vi "camera testing.vi"() -> ()   [LabVIEW 2014]
uses:
  <vilib>/vision/Vision Builder AI/API.llb/IVB Interface - VBAI Version.ctl
  <vilib>/Instr/_visa.llb/VISA Configure Serial Port (Instr).vi
panel:
  out "y-position 3":dbl
  out "x-position 3":dbl
  out "y-position 2":dbl
  out "x-position 2":dbl
  out "y-position 1":dbl
  out "XY Graph":cluster{dbl[], dbl[]}(graph)
  out "x-position 1":dbl
  out "Velocity array":dbl[][](array[numeric])
  out "Position array":dbl[][](array[numeric]) format="%#_8g"
  in  "stop":bool
  # "y-pos"
  # "N"
  # "Time"
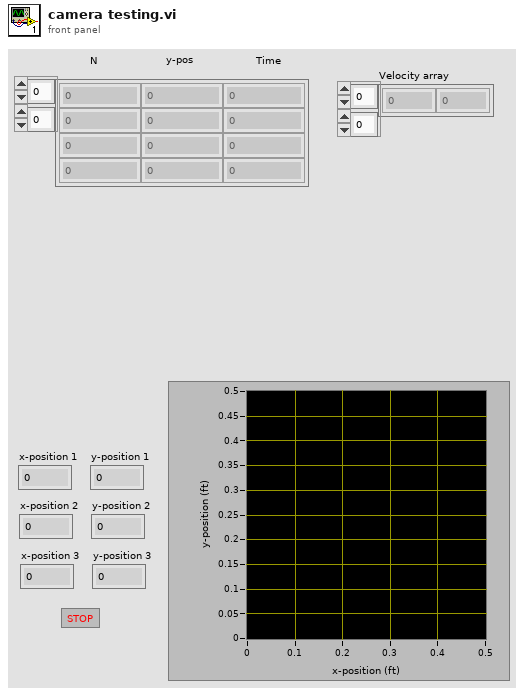
[diagram p1: front panel]
types:
  T1 = typedef "IVB Interface - VBAI Version.ctl" = u16
  T2 = typedef "VBAIInterface.ctl" = refnum<k21>
  T3 = typedef "IMAQ Image.ctl" = refnum<image>
  T4 = cluster{"PASS/FAIL Flag":bool, "Numeric Measurement":dbl, "String Measurement":string, "Report Text":string}[]
  T5 = cluster{"PASS/FAIL Flag":bool, "Numeric Measurement":dbl, "String Measurement":string, "Report Text":string}
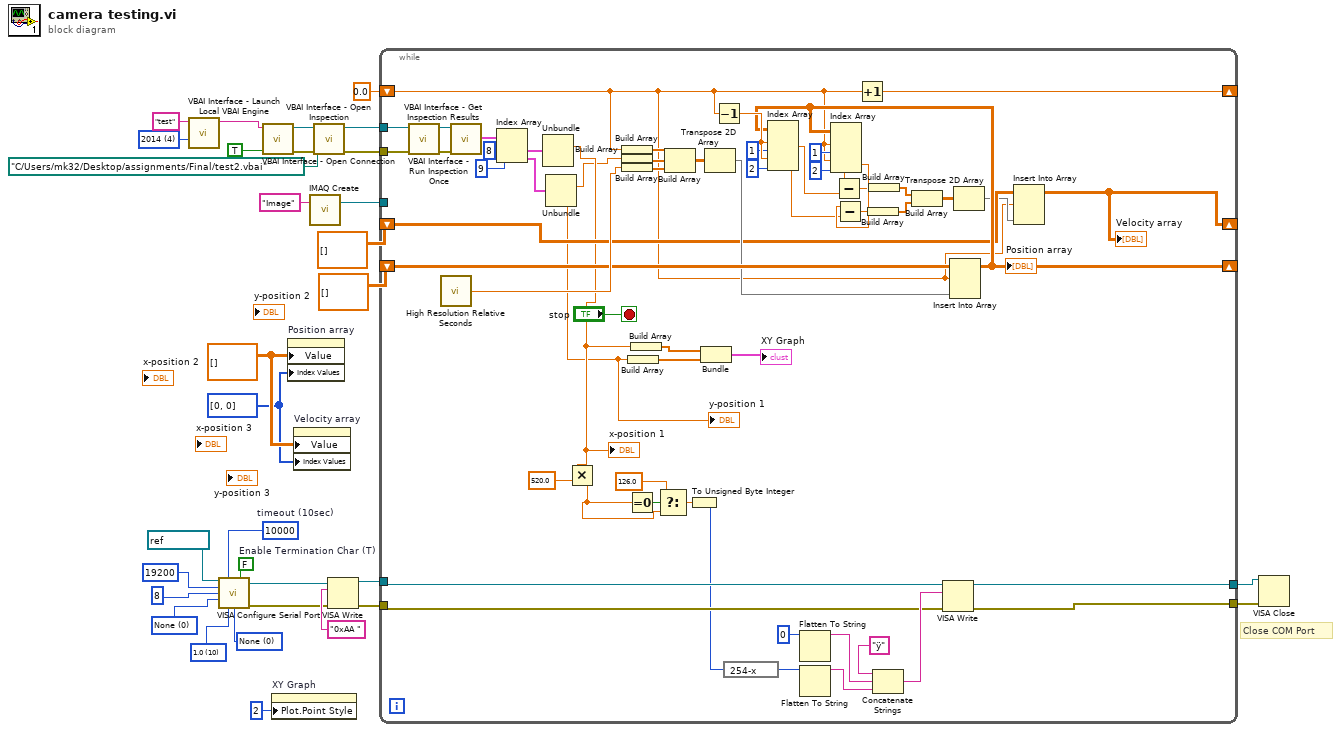
[diagram p0: block diagram]
diagram:
  w8 = u16 0 items=["None"=0, "XON/XOFF"=1, "RTS/CTS"=2, "DTR/DSR"=4] ("flow control")
  w9 = u16 10 items=["1.0"=10, "1.5"=15, "2.0"=20] ("stop bits")
  w10 = u16 0 items=["None", "Odd", "Even", "Mark", "Space"] ("parity")
  w14 = FALSE  # Enable Termination Char (T)
  w15 = u32 10000  # timeout (10sec)
  w18 = u32[] [0, 0] ("Index Values")
  w19 = dbl[][] [] ("output array")
  w28 = T1 4 items=["2010", "2011", "2012", "2013", "2014"] ("Engine Version")
  # "Close COM Port"
  n1 = call <vilib>:"VBAI Interface - Launch Local VBAI Engine.vi"("Engine Version"=w28, "Local VBAI Engine Name"="test") -> ("Session Name Out"=w29:string)  [unwired: 8 in, 1 out]
  n2 = call-poly "VISA Configure Serial Port"("VISA resource name"=refnum<visa-resource-name> "COM6", "timeout (10sec)"=w15, "Enable Termination\nChar (T)"=w14, "baud rate (9600)"=u32 19200 ("baud rate"), "data bits (8)"=u16 8 ("data bits"), "parity (0:none)"=w10, "stop bits (10: 1 bit)"=w9, "flow control (0:none)"=w8) -> ("VISA resource name out"=w6:refnum<visa-resource-name>, "error out"=w7:errorcluster)  [unwired: 1 in, 5 out]
  n3 = call <vilib>:"VBAI Interface - Open Connection.vi"("Force Connection (False)"=TRUE, "Session In"=w29) -> ("error out"=w27:errorcluster, "Session Out"=w26:T2)  [unwired: 8 in]
  n4 = property on="XY Graph" class="XYGraph (strict)"("Plot.Point Style"=u8 2) -> ()  [unwired: 2 in, 2 out]
  n5 = property on="Position array" class="Arr (strict)"("Value"=w19, "Index Values"=w18) -> ()  [unwired: 2 in, 2 out]
  n6 = property on="Velocity array" class="Arr (strict)"("Value"=w19, "Index Values"=w18) -> ()  [unwired: 2 in, 2 out]
  n7 = call "IMAQ Create"("Image Name"="Image") -> ("New Image"=w22:T3)  [unwired: 4 in, 1 out]
  n8 = call <vilib>:"VBAI Interface - Open Inspection.vi"("error in"=w27, "Path"=path "C:/Users/mk32/Desktop/assignments/Final/test2.vbai", "Session In"=w26) -> ("error out"=w23:errorcluster, "Session Out"=w24:T2)  [unwired: 7 in]
  n9 = VISA Write(VISA resource name=w6, write buffer="0xAA ", error in (no error)=w7) -> (VISA resource name out=w5:refnum<visa-resource-name>, error out=w4:errorcluster)  [unwired: 1 out]
  n10 = while {
    tunnel: w24 -> [w88]
    tunnel: w23 -> [w89]
    tunnel: w22 -> [_]
    shift-right: [w83] -> _
    shift-left: 0.0 ("Numeric Measurement") -> [w58]
    shift-right: [w61] -> _
    shift-left: dbl[][] [] ("appended array") -> [w77]
    shift-right: [w57] -> _
    shift-left: dbl[][] [] ("appended array") -> [w60]
    tunnel: w5 -> [w49]
    tunnel: w4 -> [w48]
    tunnel: [w47] -> w3
    tunnel: [w46] -> w2
    stop <- "stop" stop-if-true
    n11 = call <vilib>:"VBAI Interface - Run Inspection Once.vi"("error in"=w89, "Session In"=w88) -> ("error out"=w87:errorcluster, "Session Out"=w86:T2)  [unwired: 8 in]
    n12 = call <vilib>:"High Resolution Relative Seconds.vi"() -> ("relative seconds"=w82:dbl)
    n13 = call <vilib>:"VBAI Interface - Get Inspection Results.vi"("error in"=w87, "Session In"=w86) -> ("Step Results"=w85:T4)  [unwired: 3 in, 6 out]
    n14 = Index Array(array=w85, index #1=8 ("index"), index #2=9 ("index")) -> (element #1=w56:T5, element #2=w54:T5)
    n15 = Unbundle(w56) -> ("Numeric Measurement"=w41:dbl)  [unwired: 3 out]
    "x-position 1" <- w41
    n16 = Unbundle(w54) -> ("Numeric Measurement"=w33:dbl)  [unwired: 3 out]
    "y-position 1" <- w33
    n17 = Multiply(x=w41, y=520.0) -> (x*y=w39:dbl)
    n18 = Build Array(w58) -> (w81:dbl[])
    n19 = Build Array(w33) -> (w80:dbl[])
    n20 = Build Array(w82) -> (w79:dbl[])
    n21 = Equal To 0?(x=w39) -> (x = 0?=w42:bool)
    n22 = Build Array(w33) -> (w45:dbl[])
    n23 = Build Array(w41) -> (w44:dbl[])
    n24 = Select(t=126.0, s=w42, f=w39) -> (s? t:f=w36:dbl)
    n25 = Build Array(w81, w80, w79) -> (w78:dbl[][])
    n26 = To Unsigned Byte Integer(number=w36) -> (unsigned 8bit integer=w35:u8)
    n27 = Bundle(w44, w45) -> (→"XY Graph":cluster{dbl[], dbl[]})  [unwired: 1 in]
    n28 = Transpose 2D Array(2D array=w78) -> (transposed array=w62:dbl[][])
    n29 = Decrement(x=w58) -> (x-1=w76:dbl)
    n30 = expression code="254-x"(w35) -> (w34:u8)
    n31 = Flatten To String(anything=u8 0 ("y")) -> (data string=w52:string)  [unwired: 1 in, 4 out]
    n32 = Flatten To String(anything=w34) -> (data string=w51:string)  [unwired: 1 in, 4 out]
    n33 = Increment(x=w58) -> (x+1=w83:dbl)
    n34 = Concatenate Strings("ÿ", w52, w51) -> (w50:string)
    n35 = VISA Write(VISA resource name=w49, write buffer=w50, error in (no error)=w48) -> (VISA resource name out=w47:refnum<visa-resource-name>, error out=w46:errorcluster)  [unwired: 1 out]
    n36 = Insert Into Array(array=w77, index (row)=w58, new element=w62) -> (w61:dbl[][])  [unwired: 1 in]
    "Position array" <- w61
    n37 = Index Array(array=w61, index (row) #1=w76, index (col) #1=1 ("disabled index (col)"), index (row) #2=w76, index (col) #2=2 ("disabled index (col)")) -> (element #1=w71:dbl, element #2=w68:dbl)
    n38 = Index Array(array=w61, index (row) #1=w58, index (col) #1=1 ("disabled index (col)"), index (row) #2=w58, index (col) #2=2 ("disabled index (col)")) -> (element #1=w70:dbl, element #2=w69:dbl)
    n39 = Subtract(x=w70, y=w71) -> (x-y=w67:dbl)
    n40 = Subtract(x=w69, y=w68) -> (x-y=w66:dbl)
    n41 = Build Array(w66) -> (w64:dbl[])
    n42 = Build Array(w67) -> (w65:dbl[])
    n43 = Build Array(w65, w64) -> (w63:dbl[][])
    n44 = Transpose 2D Array(2D array=w63) -> (transposed array=w59:dbl[][])
    n45 = Insert Into Array(array=w60, index (row)=w58, new element=w59) -> (w57:dbl[][])  [unwired: 1 in]
    "Velocity array" <- w57
  }
  n46 = VISA Close(VISA resource name=w3, error in (no error)=w2) -> ()  [unwired: 1 out]
